vi "Industrial Controller.vi"(8 "error in (no error)":errorcluster, 11 "Node Ptr":T1 format="%.0x") -> (0 "error out":errorcluster)   [LabVIEW 2019, in "Control Addon System Explorer.lvlib"]
uses:
  Control Addon System Explorer.lvlib
  <vilib>/NI VeriStand/Custom Device API/Custom Device Item Ref.ctl
  NationalInstruments.VeriStand.SystemStorageUI
  Types/Action.ctl
  Addon Shared/SubVIs/Constants.vi
  <vilib>/NI VeriStand/Custom Device API/NI VeriStand - Get Item Property.vi
  <vilib>/NI VeriStand/Custom Device API/Get Item Property (Double).vi
  <vilib>/NI VeriStand/Custom Device API/Get Item Property (Boolean).vi
  <vilib>/NI VeriStand/Custom Device API/NI VeriStand - Set Item Property.vi
  <vilib>/NI VeriStand/Custom Device API/Set Item Property (Double).vi
  <vilib>/NI VeriStand/Custom Device API/Set Item Property (Boolean).vi
  <vilib>/NI VeriStand/UI Controls/Single Node Browser/Register Callbacks.vi
  <vilib>/NI VeriStand/Custom Device Tools/Custom Device Utility Library/NI VeriStand - Search for Item.vi
  <vilib>/NI VeriStand/Custom Device Tools/Custom Device Utility Library/NI VeriStand - Search for Item by GUID.vi
  <vilib>/NI VeriStand/Custom Device API/NI VeriStand - Add Custom Device Channel.vi
  <vilib>/NI VeriStand/Custom Device API/NI VeriStand - Remove Custom Device Item.vi
  <vilib>/NI VeriStand/Custom Device API/Custom Device API.lvlib
  Addon Shared/Control Addon Shared.lvlib
panel:
  in  "Description":string
  in  "Header 4":cluster{"Section Name":string}={"Section Name"="Setpoint Signal Settings"}
  in  "Header 3":cluster{"Section Name":string}={"Section Name"="Output Signal Settings"}
  in  "Header 2":cluster{"Section Name":string}={"Section Name"="Feedback Signal Settings"}
  in  "Setpoint Min":dbl caption="Setpoint Min (EU)"
  in  "Setpoint Max":dbl caption="Setpoint Max (EU)"
  in  "Output Min":dbl caption="Deactivated Level (EU)"
  in  "Output Max":dbl caption="Activated Level (EU)"
  in  "Setpoint":refnum<k24>(container)
  in  "Use External Setpoint":bool
  in  "Output":refnum<k24>(container)
  in  "Feedback":refnum<k24>(container)
  in  "SHDocVw.IWebBrowser":refnum<k7>(container)
  in  "Header":cluster{"Section Name":string}={"Section Name"="Custom Device Item Settings"}
  in  "Name":string
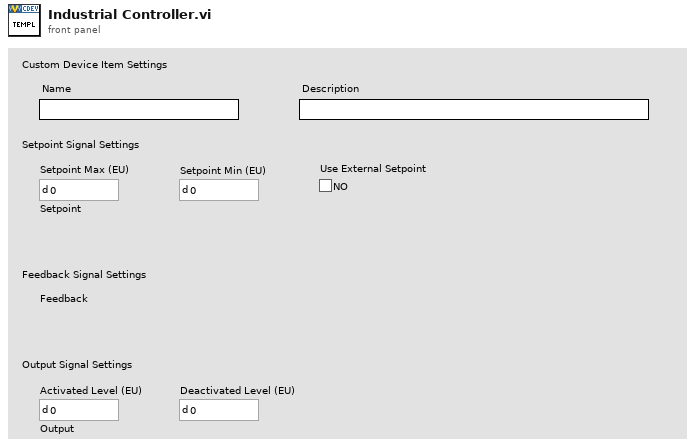
[diagram p1: front panel]
types:
  T1 = typedef "Custom Device API.lvlib/Custom Device Item Ref.ctl" = u64
  T2 = typedef "Control Addon System Explorer.lvlib/Action.ctl" = enum16{"Get", "Set"}
  T3 = typedef "Control Addon Shared.lvlib/Controller Settings.ctl" = cluster{"Output Max":dbl, "Output Min":dbl, "Setpoint Max":dbl, "Setpoint Min":dbl, "Use External Setpoint":bool, "Output Rate Limiter":dbl}
  T4 = typedef "Control Addon System Explorer.lvlib/PID Controller Channel Browser Refs.ctl" = cluster{"Output":refnum<user-event>, "Setpoint":refnum<user-event>, "Feedback":refnum<user-event>}
  T5 = typedef "Custom Device API.lvlib/Custom Device Item Info.ctl" = cluster{"Name":string, "Is Channel":bool, "GUID":string, "Is Waveform":bool}
  T6 = typedef "Custom Device API.lvlib/Custom Device Commands.ctl" = enum16{"Default", "Item renamed", "Shutdown", "Dynamic button pressed"}
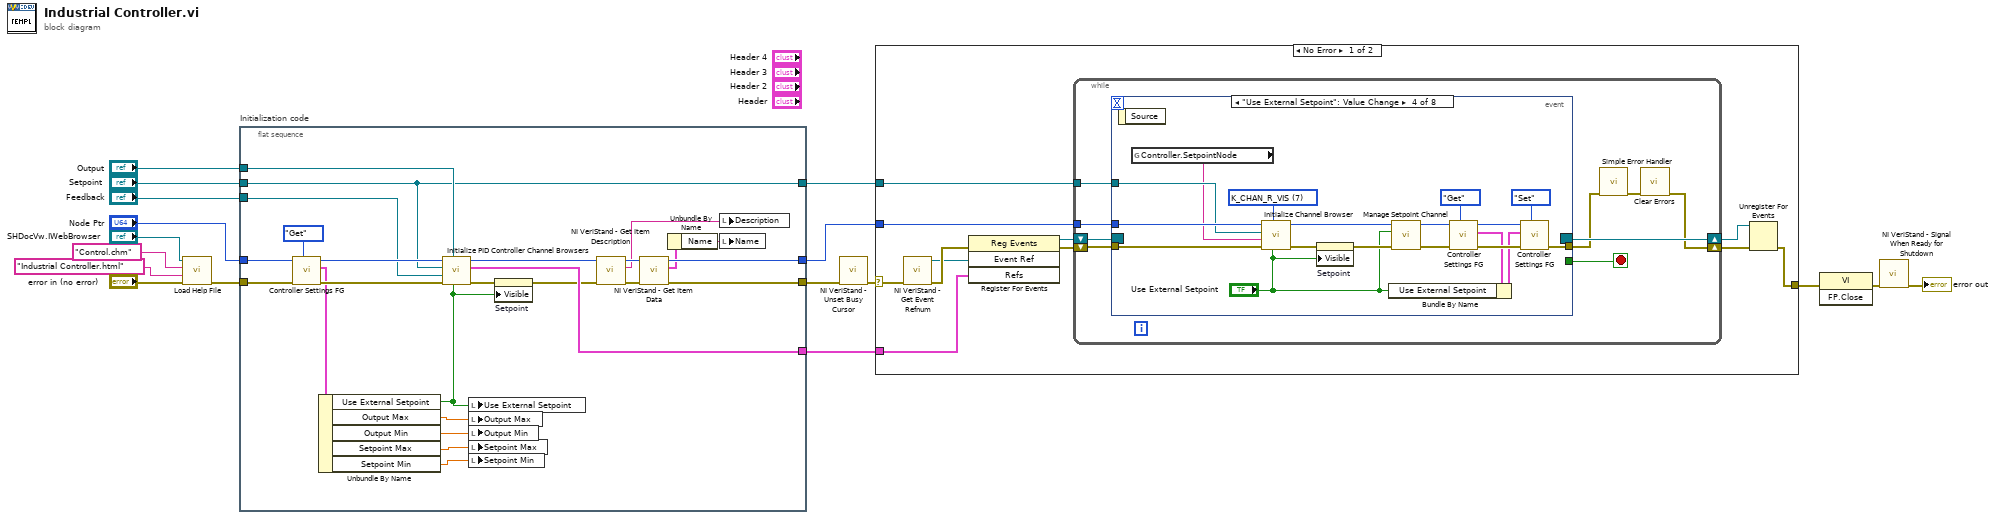
[diagram p0: block diagram]
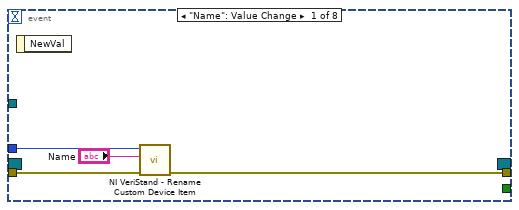
[diagram p2: hidden frame]
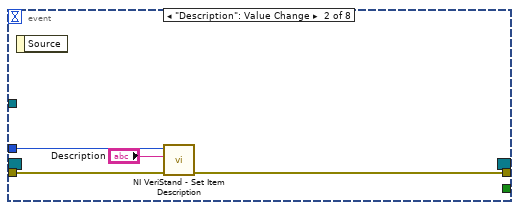
[diagram p3: hidden frame]
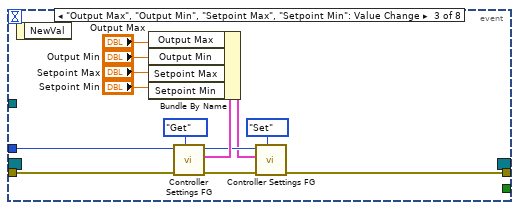
[diagram p4: hidden frame]
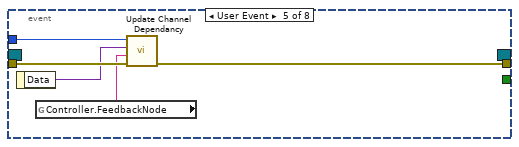
[diagram p5: hidden frame]
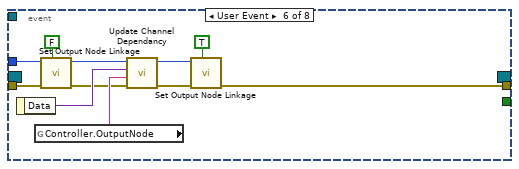
[diagram p6: hidden frame]
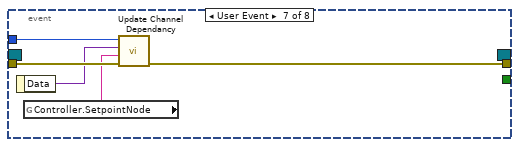
[diagram p7: hidden frame]
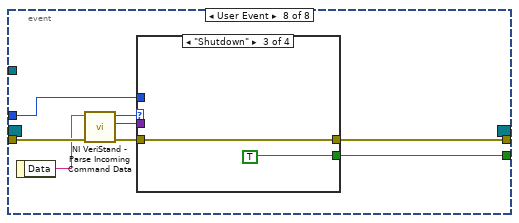
[diagram p8: hidden frame]
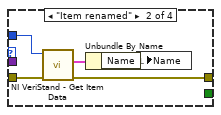
[diagram p10: hidden frame]
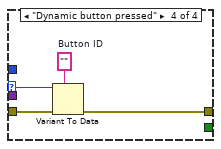
[diagram p11: hidden frame]
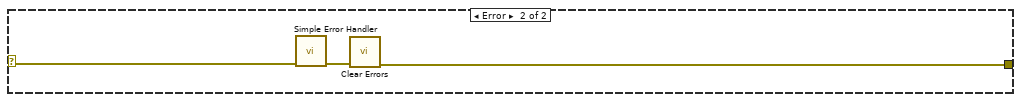
[diagram p12: hidden frame]
diagram:
  n1 = call "Load Help File.vi"("error in (no error)"="error in (no error)", "HTML File"="Industrial Controller.html", "Main CHM File"="Control.chm", "SHDocVw.IWebBrowser2"="SHDocVw.IWebBrowser") -> ("error out"=w9:errorcluster)  [unwired: 7 in]
  n2 = flat-sequence "Initialization code" {
    tunnel: w9 -> [w34]
    tunnel: "Node Ptr" -> [w33]
    tunnel: [w36] -> w13
    tunnel: [w42] -> w11
    tunnel: [w24] -> w5
    tunnel: [w19] -> w4
    tunnel: "Output" -> [w20]
    tunnel: "Setpoint" -> [w19]
    tunnel: "Feedback" -> [w18]
    frame #0 {
      n3 = call "Controller Settings FG.vi"("Action"=Action."Get", "error in (no error)"=w34, "Node Ptr"=w33) -> ("error out"=w31:errorcluster, "Controller Settings"=w29:T3, "Item Ref out"=w32:T1)  [unwired: 6 in]
      n4 = Unbundle By Name(w29) -> ("Use External Setpoint"=w21:bool, "Output Max"=w28:dbl, "Output Min"=w27:dbl, "Setpoint Max"=w26:dbl, "Setpoint Min"=w25:dbl)
      n5 = call "Initialize PID Controller Channel Browsers.vi"("Use External Setpoint"=w21, "Output"=w20, "error in (no error)"=w31, "Feedback"=w18, "Setpoint in"=w19, "Item Ref in"=w32) -> ("error out"=w23:errorcluster, "Refs"=w24:T4, "Item Ref out"=w35:T1)  [unwired: 3 in]
      n6 = local write "Use External Setpoint"(w21) -> ()
      n7 = local write "Output Max"(w28) -> ()
      n8 = local write "Output Min"(w27) -> ()
      n9 = local write "Setpoint Max"(w26) -> ()
      n10 = local write "Setpoint Min"(w25) -> ()
      n11 = property on="Setpoint" class="AXCont"(error in=w23, "Visible"=w21) -> (error out=w22:errorcluster)  [unwired: 1 in, 1 out]
      n12 = call <vilib>:"NI VeriStand - Get Item Description.vi"("error in (no error)"=w22, "Item Ref in"=w35) -> ("error out"=w39:errorcluster, "Description"=w40:string, "Item Ref out"=w41:T1)  [unwired: 7 out]
      n13 = call <vilib>:"NI VeriStand - Get Item Data.vi"("error in (no error)"=w39, "Item Ref in"=w41) -> ("error out"=w36:errorcluster, "Item Info"=w38:T5, "Item Ref out"=w42:T1)  [unwired: 7 out]
      n14 = Unbundle By Name(w38) -> ("Name"=w37:string)
      n15 = local write "Description"(w40) -> ()
      n16 = local write "Name"(w37) -> ()
    }
  }
  n17 = call <vilib>:"NI VeriStand - Unset Busy Cursor.vi"("error in (no error)"=w13) -> ("error out"=w12:errorcluster)  [unwired: 10 out]
  n18 = case shown="No Error" w12 {
    selector: w12 -> [w45 w145]
    tunnel: [w50 w143] -> w17
    tunnel: w11 -> [w46 _]
    tunnel: w5 -> [w43 _]
    tunnel: w4 -> [w44 _]
    frame No Error {
      n19 = call <vilib>:"NI VeriStand - Get Event Refnum.vi"("error in (no error)"=w45) -> ("error out"=w53:errorcluster, "Event Ref"=w49:refnum<user-event>)  [unwired: 9 out]
      n20 = register-events(error in=w53, w49, w43) -> (reference out=w47:refnum<event-registration>, error out=w48:errorcluster)  [unwired: 1 in]
      n21 = while {
        tunnel: w46 -> [w58]
        shift-right: [w55] -> w51
        shift-left: w48 -> [w61]
        shift-right: [w62] -> w52
        shift-left: w47 -> [w60]
        tunnel: w44 -> [w54]
        stop <- w59 stop-if-true
        n22 = event shown="[3] \"Use External Setpoint\": Value Change" {
          selector: w60 -> [_ _ _ _ _ _ _ _]
          dyn-events: [_ _ _ _ _ _ _ _] -> w62
          timeout: _ -> [_ _ _ _ _ _ _ _]
          tunnel: w61 -> [w66 w69 w82 w94 w106 w111 w122 w130]
          tunnel: [_ _ _ _ _ _ _ w126] -> w59
          tunnel: [w65 w68 w75 w97 w105 w107 w121 w125] -> w57
          tunnel: w58 -> [w64 w70 w81 w93 w104 w110 w120 w124]
          tunnel: w54 -> [_ _ _ w91 _ _ _ _]
          event "Name": Value Change {
            n23 = event-data() -> ()  [unwired: 2 out]
            n24 = call <vilib>:"NI VeriStand - Rename Custom Device Item.vi"("error in (no error)"=w66, "New Name"="Name", "Item Ref in"=w64) -> ("error out"=w65:errorcluster)  [unwired: 1 in, 7 out]
          }
          event "Description": Value Change {
            n25 = event-data() -> ()  [unwired: 2 out]
            n26 = call <vilib>:"NI VeriStand - Set Item Description.vi"("error in (no error)"=w69, "Description"="Description", "Item Ref in"=w70) -> ("error out"=w68:errorcluster)  [unwired: 8 out]
          }
          event "Output Max", "Output Min", "Setpoint Max", "Setpoint Min": Value Change {
            n27 = event-data() -> ()  [unwired: 2 out]
            n28 = call "Controller Settings FG.vi"("Action"=Action."Get", "error in (no error)"=w82, "Node Ptr"=w81) -> ("error out"=w77:errorcluster, "Controller Settings"=w80:T3, "Item Ref out"=w78:T1)  [unwired: 6 in]
            n29 = Bundle By Name(cluster=w80, "Output Max"="Output Max", "Output Min"="Output Min", "Setpoint Max"="Setpoint Max", "Setpoint Min"="Setpoint Min") -> (w76:T3)
            n30 = call "Controller Settings FG.vi"("Action"=Action."Set", "error in (no error)"=w77, "Controller Settings"=w76, "Node Ptr"=w78) -> ("error out"=w75:errorcluster)  [unwired: 5 in, 2 out]
          }
          event "Use External Setpoint": Value Change {
            w92 = u8 7 items=["K_CHAN_R", "K_CHAN_W", "K_CHAN_RW", "K_CHAN_VOLT", "K_CHAN_FAULT", "K_ALL", "K_CUSTOM", "K_CHAN_R_VIS", "K_CHAN_W_VIS", "K_CHAN_RW_VIS", "K_CHAN_VOLT_VIS", "K_CHAN_FAULT_VIS"] ("DisplayFilter")
            n31 = event-data() -> ()  [unwired: 2 out]
            n32 = global read "Constants.vi" "Controller.SetpointNode"() -> (w84:string)
            n33 = call "Initialize Channel Browser.vi"("Use Channel?"="Use External Setpoint", "DisplayFilter"=w92, "error in (no error)"=w94, "NodeName"=w84, "Browser Ref"=w91, "Item Ref in"=w93) -> ("error out"=w87:errorcluster, "Item Ref out"=w90:T1)  [unwired: 3 in, 1 out]
            n34 = property on="Setpoint" class="AXCont"(error in=w87, "Visible"="Use External Setpoint") -> (error out=w86:errorcluster)  [unwired: 1 in, 1 out]
            n35 = call "Manage Setpoint Channel.vi"("error in (no error)"=w86, "Use External Setpoint"="Use External Setpoint", "Node Ptr"=w90) -> ("error out"=w88:errorcluster, "Node Ptr out"=w89:T1)  [unwired: 7 in]
            n36 = call "Controller Settings FG.vi"("Action"=Action."Get", "error in (no error)"=w88, "Node Ptr"=w89) -> ("error out"=w98:errorcluster, "Controller Settings"=w96:T3, "Item Ref out"=w99:T1)  [unwired: 6 in]
            n37 = Bundle By Name(cluster=w96, "Use External Setpoint"="Use External Setpoint") -> (w95:T3)
            n38 = call "Controller Settings FG.vi"("Action"=Action."Set", "error in (no error)"=w98, "Controller Settings"=w95, "Node Ptr"=w99) -> ("error out"=w97:errorcluster)  [unwired: 5 in, 2 out]
          }
          event User Event {
            n39 = event-data() -> ("Data"=w103:variant)  [unwired: 1 out]
            n40 = global read "Constants.vi" "Controller.FeedbackNode"() -> (w102:string)
            n41 = call "Update Channel Dependancy.vi"("error in (no error)"=w106, "NodeName"=w102, "Data"=w103, "Item Ref in"=w104) -> ("error out"=w105:errorcluster)  [unwired: 6 in, 1 out]
          }
          event User Event {
            n42 = event-data() -> ("Data"=w117:variant)  [unwired: 1 out]
            n43 = global read "Constants.vi" "Controller.OutputNode"() -> (w116:string)
            n44 = call "Set Output Node Linkage.vi"("Add?"=FALSE, "error in"=w111, "Section Ref in"=w110) -> ("error out"=w109:errorcluster, "Item Ref out"=w108:T1)  [unwired: 7 in]
            n45 = call "Update Channel Dependancy.vi"("error in (no error)"=w109, "NodeName"=w116, "Data"=w117, "Item Ref in"=w108) -> ("error out"=w115:errorcluster, "Item Ref out"=w114:T1)  [unwired: 6 in]
            n46 = call "Set Output Node Linkage.vi"("Add?"=TRUE, "error in"=w115, "Section Ref in"=w114) -> ("error out"=w107:errorcluster)  [unwired: 7 in, 1 out]
          }
          event User Event {
            n47 = event-data() -> ("Data"=w119:variant)  [unwired: 1 out]
            n48 = global read "Constants.vi" "Controller.SetpointNode"() -> (w118:string)
            n49 = call "Update Channel Dependancy.vi"("error in (no error)"=w122, "NodeName"=w118, "Data"=w119, "Item Ref in"=w120) -> ("error out"=w121:errorcluster)  [unwired: 6 in, 1 out]
          }
          event User Event {
            n50 = event-data() -> ("Data"=w129:string)  [unwired: 1 out]
            n51 = call <vilib>:"NI VeriStand - Parse Incoming Command Data.vi"("error in (no error)"=w130, "Incoming data"=w129) -> ("error out"=w128:errorcluster, "Outgoing data"=w123:variant, "Action"=w127:T6)  [unwired: 7 out]
            n52 = case shown="\"Shutdown\"" w127 {
              tunnel: w128 -> [w131 w136 w137 w142]
              tunnel: [_ _ TRUE _] -> w126
              tunnel: [w131 w133 w137 w139] -> w125
              tunnel: w124 -> [_ w135 _ _]
              tunnel: w123 -> [_ _ _ w141]
              frame "Default", Default {
              }
              frame "Item renamed" {
                n53 = call <vilib>:"NI VeriStand - Get Item Data.vi"("error in (no error)"=w136, "Item Ref in"=w135) -> ("error out"=w133:errorcluster, "Item Info"=w134:T5)  [unwired: 8 out]
                n54 = Unbundle By Name(w134) -> ("Name"=w132:string)
                n55 = local write "Name"(w132) -> ()
              }
              frame "Shutdown" {
              }
              frame "Dynamic button pressed" {
                w140 = ""  # Button ID
                n56 = Variant To Data(error in=w142, type=w140, Variant=w141) -> (error out=w139:errorcluster)  [unwired: 1 out]
              }
            }
          }
        }
        n57 = call <vilib>:"Simple Error Handler.vi"("error in (no error)"=w57) -> ("error out"=w56:errorcluster)  [unwired: 1 in, 7 out]
        n58 = call <vilib>:"Clear Errors.vi"("error in (no error)"=w56) -> ("error out"=w55:errorcluster)  [unwired: 1 in, 5 out]
      }
      n59 = Unregister For Events(event registration refnum=w52, error in=w51) -> (error out=w50:errorcluster)
    }
    frame Error {
      n60 = call <vilib>:"Simple Error Handler.vi"("error in (no error)"=w145) -> ("error out"=w144:errorcluster)  [unwired: 1 in, 7 out]
      n61 = call <vilib>:"Clear Errors.vi"("error in (no error)"=w144) -> ("error out"=w143:errorcluster)  [unwired: 1 in, 5 out]
    }
  }
  n62 = invoke class="VI" method="FP.Close"(error in=w17) -> (error out=w16:errorcluster)  [unwired: 2 in, 2 out]
  n63 = call <vilib>:"NI VeriStand - Signal When Ready for Shutdown.vi"("error in (no error)"=w16) -> ("error out"=→"error out":errorcluster)  [unwired: 10 out]
